vi "Subvi mem address.vi"(9 "Count":u16) -> (0 "Gating out":bool, 1 "Addres":u16)   [LabVIEW 2017]
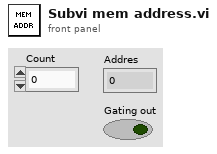
[diagram p1: front panel]
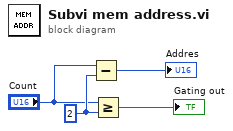
[diagram p0: block diagram]
diagram:
  w4 = u16 2 ("y")
  n1 = Subtract(x="Count", y=w4) -> (x-y=→"Addres":u16)
  n2 = Greater Or Equal?(x="Count", y=w4) -> (x >= y?=→"Gating out":bool)
